vi "SL2_AD_DLL_Phoibos_Initialize.vi"(4 "error in":errorcluster, 5 "detectorId":string, 6 "analyzerId":string, 7 "dll_path":path) -> (0 "error out":errorcluster, 1 "pHandle":u32, 3 "path out":path)   [LabVIEW 2020]
uses:
  DEFINITIONS/DEF_T_error_enum.ctl
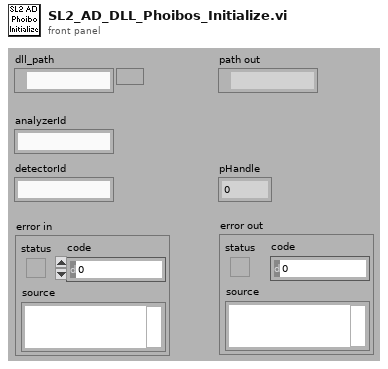
[diagram p1: front panel]
types:
  T1 = typedef "DEF_T_error_enum.ctl" = u32
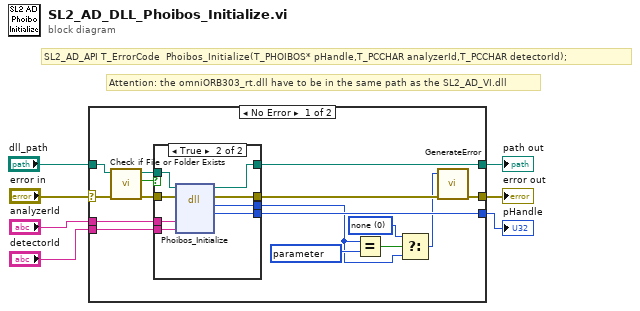
[diagram p0: block diagram]
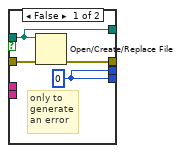
[diagram p2: hidden frame]
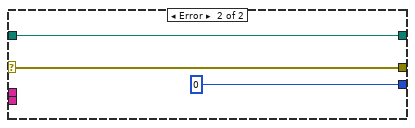
[diagram p3: hidden frame]
diagram:
  # "SL2_AD_API T_ErrorCode  Phoibos_Initialize(T_PHOIBOS* pHandle,T_PCCHAR analyzerId,T_PCCHAR detectorId);"
  # "Attention: the omniORB303_rt.dll have to be in the same path as the SL2_AD_VI.dll"
  n1 = case shown="No Error" "error in" {
    selector: "error in" -> [w22 w38]
    tunnel: [w16 w38] -> w7
    tunnel: [w23 w37] -> w6
    tunnel: "dll_path" -> [w21 w37]
    tunnel: "analyzerId" -> [w20 _]
    tunnel: "detectorId" -> [w19 _]
    tunnel: [w18 u32 0 ("pHandle")] -> w1
    frame No Error {
      w12 = T1 0 items=["none"=0, "busy"=65536, "error"=131072, "parameter"=262144, "locked"=524288, "sync"=1048576, "connection"=2097152, "internal"=4194304, "end_of_data"=8388608] ("error_code")
      w15 = T1 262144 items=["none"=0, "busy"=65536, "error"=131072, "parameter"=262144, "locked"=524288, "sync"=1048576, "connection"=2097152, "internal"=4194304, "end_of_data"=8388608] ("error_code")
      n2 = call <vilib>:"Check if File or Folder Exists.vi"("error in (no error)"=w22, "path"=w21) -> ("error out"=w10:errorcluster, "file or folder exists?"=w8:bool, "dup path"=w9:path)  [unwired: 7 in]
      n3 = case shown="True" w8 {
        tunnel: [w27 w30] -> w17
        tunnel: [w25 w29] -> w23
        tunnel: w10 -> [w26 w35]
        tunnel: w9 -> [w25 w34]
        tunnel: w20 -> [_ w33]
        tunnel: w19 -> [_ w32]
        tunnel: [w24 w31] -> w18
        tunnel: [w24 w28] -> w11
        frame False {
          w24 = u32 0 ("pHandle")
          # "only to generate an error"
          n4 = Open/Create/Replace File(file path (use dialog)=w25, error in=w26) -> (error out=w27:errorcluster)  [unwired: 4 in, 2 out]
        }
        frame True {
          n5 = dll-call lib="C:/Programme/SPECS/SpecsLab2/programming/LabView7.1/SL2_AD_VI.dll" fn="Phoibos_Initialize" label="Initilialize"(path in=w34, error in=w35, "analyzerId"=w33, "detectorId"=w32) -> (path out=w29:path, error out=w30:errorcluster, "errorcode"=w28:u32, "pHandle"=w31:u32)  [unwired: 4 in]
        }
      }
      n6 = Equal?(x=w11, y=w15) -> (x = y?=w13:bool)
      n7 = Select(t=w12, s=w13, f=w11) -> (s? t:f=w14:T1)
      n8 = call "GenerateError.vi"("error in"=w17, "error_code"=w14) -> ("error out"=w16:errorcluster)  [unwired: 9 in]
    }
    frame Error {
    }
  }
  "error out" <- w7
  "path out" <- w6
  "pHandle" <- w1
